vi "fetch_TLC.vi"(8 "error in (no error)":errorcluster, 11 "GenericToplevelComponent in":refnum<class "GenericToplevelComponent.lvclass">) -> (0 "error out":errorcluster, 3 "GenericToplevelComponent out":refnum<class "GenericToplevelComponent.lvclass">)   [LabVIEW 2010, in "GenericToplevelComponent.lvclass"]
uses:
  GenericToplevelComponent.lvclass
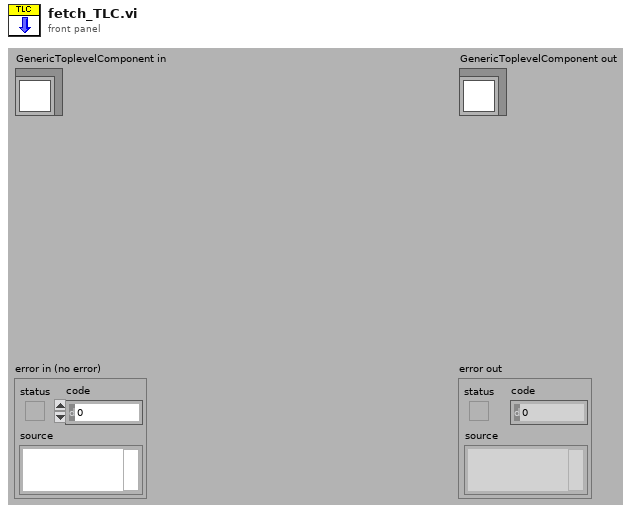
[diagram p1: front panel]
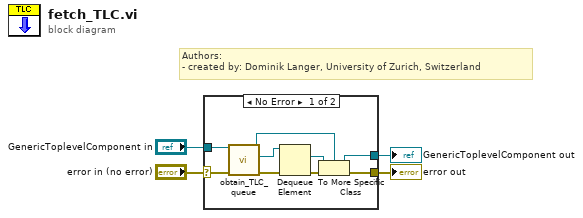
[diagram p0: block diagram]
diagram:
  # "Authors: \n- created by: Dominik Langer, University of Zurich, Switzerland"
  n1 = case shown="No Error" "error in (no error)" {
    selector: "error in (no error)" -> [w12 w15]
    tunnel: [w8 w15] -> w3
    tunnel: [w6 w14] -> w1
    tunnel: "GenericToplevelComponent in" -> [w10 w14]
    frame No Error {
      n2 = call-dynamic "obtain_TLC_queue.vi"("error in (no error)"=w12, "GenericToplevelComponent in"=w10) -> ("error out"=w13:errorcluster, "TLC queue"=w11:refnum<queue>, "GenericToplevelComponent out"=w5:refnum<class "GenericToplevelComponent.lvclass">)  [unwired: 7 in]
      n3 = Dequeue Element(queue=w11, error in (no error)=w13) -> (element=w7:refnum<class "GenericComponent.lvclass">, error out=w9:errorcluster)  [unwired: 3 out]
      n4 = To More Specific Class(target class=w5, reference=w7, error in=w9) -> (specific class reference=w6:refnum<class "GenericToplevelComponent.lvclass">, error out=w8:errorcluster)
    }
    frame Error {
    }
  }
  "error out" <- w3
  "GenericToplevelComponent out" <- w1
